vi "GetClusterValue.vi"(0 "VI Reference":refnum<vi>, 7 "Array":string[](array[string]), 11 "error in":errorcluster) -> (4 "VI Reference out":refnum<vi>, 8 "Value":variant, 15 "error out":errorcluster)   [LabVIEW 2016]
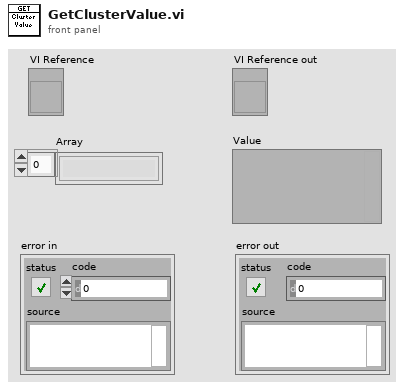
[diagram p1: front panel]
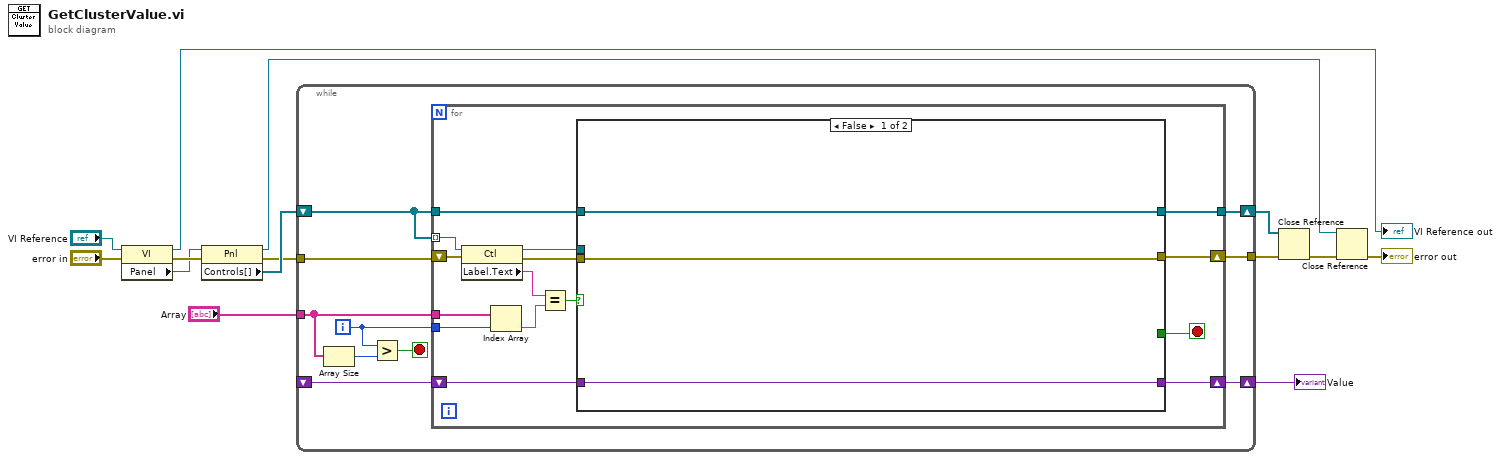
[diagram p0: block diagram]
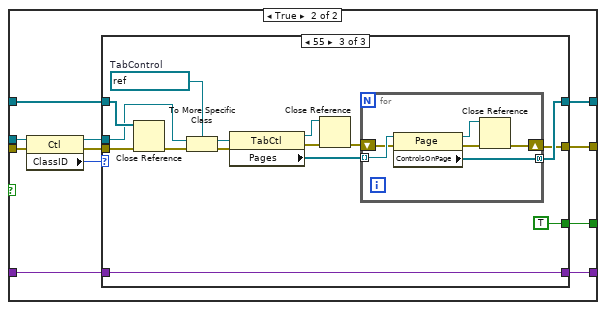
[diagram p2: hidden frame]
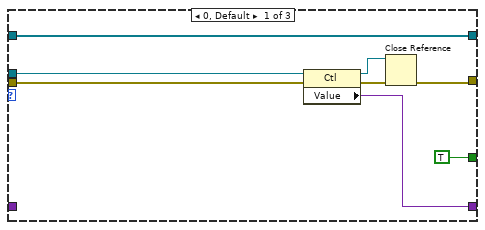
[diagram p3: hidden frame]
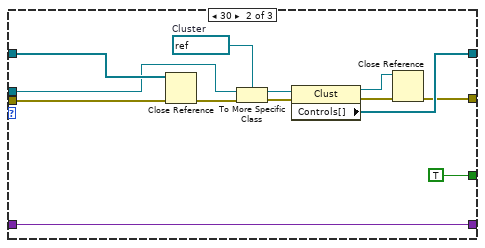
[diagram p4: hidden frame]
diagram:
  n1 = property class="VI"(reference="VI Reference", error in="error in") -> (reference out=→"VI Reference out":refnum<vi>, error out=w14:errorcluster, "Panel"=w13:refnum<vi>)
  n2 = property class="Pnl"(reference=w13, error in=w14) -> (reference out=w3:refnum<vi>, error out=w8:errorcluster, "Controls[]"=w10:refnum<vi>[])
  n3 = while {
    tunnel: "Array" -> [w20]
    shift-right: [w24] -> w4
    shift-left: w10 -> [w23]
    tunnel: w8 -> [w21]
    tunnel: [w22] -> w6
    shift-right: [w17] -> w1
    shift-left: _ -> [w15]
    i -> [w18]
    stop <- w16 stop-if-true
    n4 = Array Size(array=w20) -> (size(s)=w19:i32)
    n5 = Greater?(x=w18, y=w19) -> (0:w16:bool)
    n6 = for {
      tunnel: w23 -> [w39] mode=indexing
      tunnel: w20 -> [w37]
      tunnel: [w31] -> w24
      tunnel: w18 -> [w33]
      tunnel: w23 -> [w32]
      shift-right: [w29] -> w22
      shift-left: w21 -> [w28]
      shift-right: [w27] -> w17
      shift-left: w15 -> [w25]
      stop <- w26 stop-if-true
      n7 = property class="Ctl"(reference=w39, error in=w28) -> (reference out=w34:refnum<vi>, error out=w30:errorcluster, "Label.Text"=w38:string)
      n8 = Index Array(array=w37, index=w33) -> (element=w36:string)
      n9 = Equal?(x=w38, y=w36) -> (x = y?=w35:bool)
      n10 = case shown="False" w35 {
        tunnel: w34 -> [_ w53]
        tunnel: [w41 w50] -> w31
        tunnel: w32 -> [w41 w49]
        tunnel: w30 -> [w42 w47]
        tunnel: [w42 w46] -> w29
        tunnel: [_ w45] -> w26
        tunnel: [w40 w44] -> w27
        tunnel: w25 -> [w40 w43]
        frame False {
        }
        frame True {
          n11 = property class="Ctl"(reference=w53, error in=w47) -> (reference out=w51:refnum<vi>, error out=w48:errorcluster, "ClassID"=w52:u32)
          n12 = case shown="55" w52 {
            tunnel: w51 -> [w61 w64 w80]
            tunnel: [w60 w73 w85] -> w50
            tunnel: w49 -> [w60 w69 w83]
            tunnel: [TRUE TRUE TRUE] -> w45
            tunnel: w48 -> [w59 w66 w82]
            tunnel: [w57 w67 w84] -> w46
            tunnel: [w54 w62 w75] -> w44
            tunnel: w43 -> [_ w62 w75]
            frame 0, Default {
              n13 = property class="Ctl"(reference=w61, error in=w59) -> (reference out=w56:refnum<vi>, error out=w58:errorcluster, "Value"=w54:variant)
              n14 = Close Reference(reference=w56, error in (no error)=w58) -> (error out=w57:errorcluster)
            }
            frame 30 {
              w74 = refnum<vi> refnum  # Cluster
              n15 = Close Reference(reference=w69, error in (no error)=w66) -> (error out=w65:errorcluster)
              n16 = To More Specific Class(target class=w74, reference=w64, error in=w65) -> (specific class reference=w72:refnum<vi>, error out=w71:errorcluster)
              n17 = property class="Clust"(reference=w72, error in=w71) -> (reference out=w70:refnum<vi>, error out=w68:errorcluster, "Controls[]"=w73:refnum<vi>[])
              n18 = Close Reference(reference=w70, error in (no error)=w68) -> (error out=w67:errorcluster)
            }
            frame 55 {
              w89 = refnum<vi> refnum  # TabControl
              n19 = Close Reference(reference=w83, error in (no error)=w82) -> (error out=w81:errorcluster)
              n20 = To More Specific Class(target class=w89, reference=w80, error in=w81) -> (specific class reference=w88:refnum<vi>, error out=w87:errorcluster)
              n21 = property class="TabCtl"(reference=w88, error in=w87) -> (reference out=w79:refnum<vi>, error out=w78:errorcluster, "Pages"=w86:refnum<vi>[])
              n22 = Close Reference(reference=w79, error in (no error)=w78) -> (error out=w77:errorcluster)
              n23 = for {
                tunnel: w86 -> [w95] mode=indexing
                tunnel: [w94] -> w85 mode=concatenating
                shift-right: [w91] -> w84
                shift-left: w77 -> [w93]
                n24 = property class="Page"(reference=w95, error in=w93) -> (reference out=w90:refnum<vi>, error out=w92:errorcluster, "ControlsOnPage"=w94:refnum<vi>[])
                n25 = Close Reference(reference=w90, error in (no error)=w92) -> (error out=w91:errorcluster)
              }
            }
          }
        }
      }
    }
  }
  "Value" <- w1
  n26 = Close Reference(reference=w4, error in (no error)=w6) -> (error out=w2:errorcluster)
  n27 = Close Reference(reference=w3, error in (no error)=w2) -> (error out=→"error out":errorcluster)
